vi "main.vi"() -> ()   [LabVIEW 2018]
uses:
  D:/NI LabVIEW/PowerControlWithAT2/REMOTE_SEE_CONTROLLER/RemoteSeeAbleService.dll
  RemoteSeeAbleService.dll
panel:
  in  "TryParrySeeDone":bool
  in  "StartTryParrySee":bool
  in  "ShutdownDone":bool
  in  "StartShutdown":bool
  in  "IsParryable":bool
  in  "ExamineSeeDone":bool
  in  "StartExamineSee":bool
  in  "stop":bool
  in  "CheckSeeDone":bool
  in  "StartCheckSee":bool
  in  "SeeInfo":string
  in  "IsIncomplete":bool
  in  "IsSee":bool
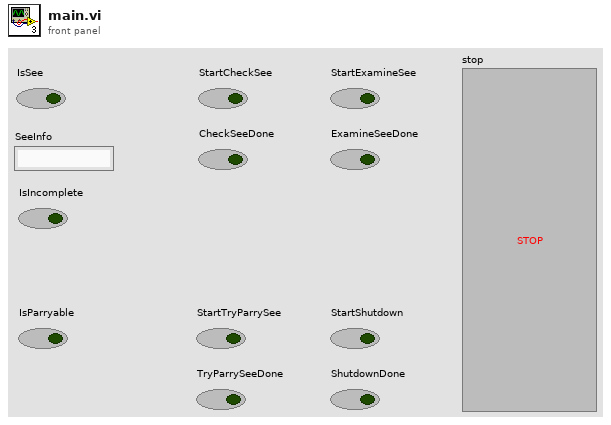
[diagram p1: front panel]
types:
  T1 = cluster{"StartCheckSee":refnum<vi>, "CheckSeeDone":refnum<vi>, "IsSee":refnum<vi>, "SeeInfo":refnum<vi>, "IsIncomplete":refnum<vi>}
  T2 = cluster{"StartExamineSee":refnum<vi>, "ExamineSeeDone":refnum<vi>, "IsSee":refnum<vi>, "SeeInfo":refnum<vi>, "IsIncomplete":refnum<vi>}
  T3 = cluster{"StartShutdown":refnum<vi>, "ShutdownDone":refnum<vi>}
  T4 = cluster{"StartTryParrySee":refnum<vi>, "TryParrySeeDone":refnum<vi>}
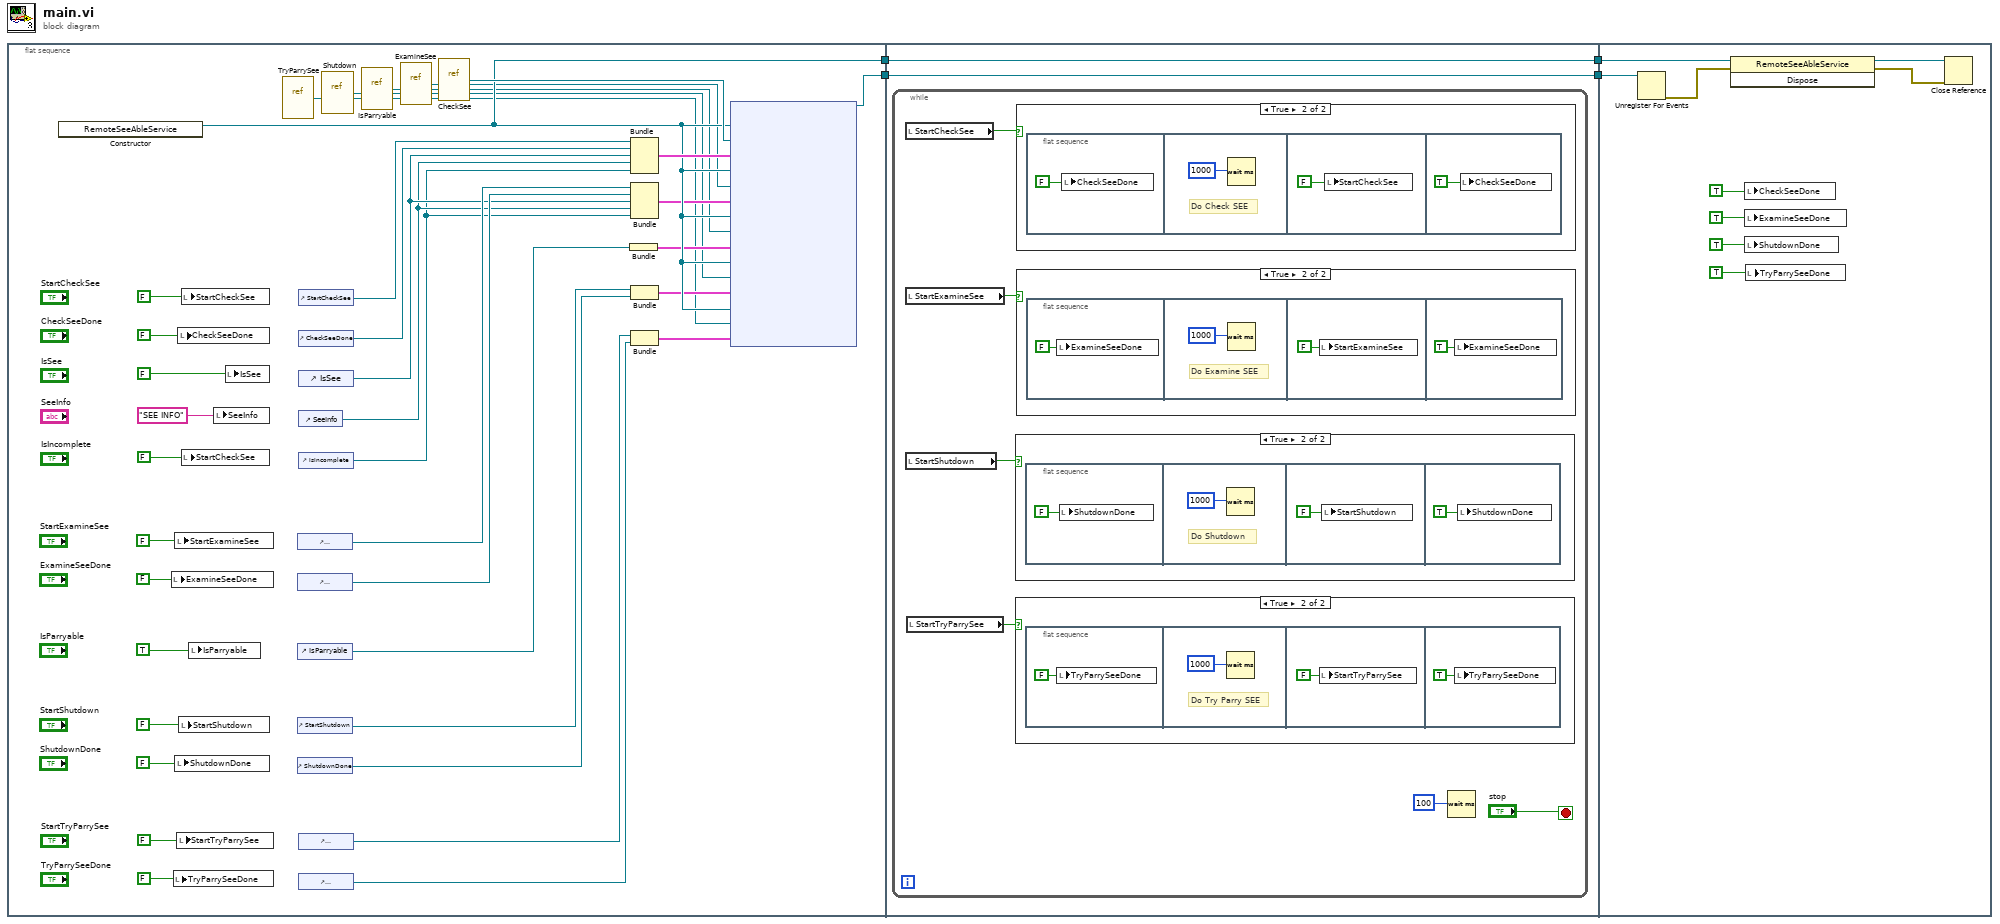
[diagram p0: block diagram]
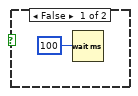
[diagram p2: hidden frame]
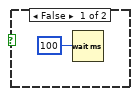
[diagram p3: hidden frame]
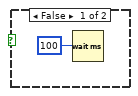
[diagram p4: hidden frame]
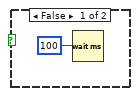
[diagram p5: hidden frame]
diagram:
  n1 = flat-sequence {
    tunnel: [w31] -> w3
    tunnel: [w30] -> w1
    tunnel: [w42] -> w4
    tunnel: w3 -> [w42]
    tunnel: [w41] -> w2
    tunnel: w1 -> [w41]
    tunnel: w4 -> [w76]
    tunnel: w2 -> [w75]
    frame #0 {
      n2 = constructor class="RemoteSeeAbleService"() -> (reference out=w31:refnum<k24>)  [unwired: 3 in, 2 out]
      n3 = local write "ExamineSeeDone"(FALSE ("StartCheckSee")) -> ()
      n4 = local write "TryParrySeeDone"(FALSE ("StartCheckSee")) -> ()
      n5 = local write "StartExamineSee"(FALSE ("StartCheckSee")) -> ()
      n6 = local write "ShutdownDone"(FALSE ("StartCheckSee")) -> ()
      n7 = local write "StartTryParrySee"(FALSE ("StartCheckSee")) -> ()
      n8 = local write "CheckSeeDone"(FALSE ("StartCheckSee")) -> ()
      n9 = local write "StartShutdown"(FALSE ("StartCheckSee")) -> ()
      n10 = local write "StartCheckSee"(FALSE ("StartCheckSee")) -> ()
      n11 = local write "StartCheckSee"(FALSE ("StartCheckSee")) -> ()
      n12 = local write "IsParryable"(TRUE ("StartCheckSee")) -> ()
      n13 = local write "SeeInfo"("SEE INFO" ("SeeInfo")) -> ()
      n14 = local write "IsSee"(FALSE ("StartCheckSee")) -> ()
      n15 = vi-ref "TryParrySee.vi"() -> ("vi reference"=w5:refnum<vi>)
      n16 = control-ref of="StartExamineSee"() -> (w27:refnum<vi>)
      n17 = control-ref of="ExamineSeeDone"() -> (w26:refnum<vi>)
      n18 = control-ref of="IsParryable"() -> (w20:refnum<vi>)
      n19 = control-ref of="StartShutdown"() -> (w16:refnum<vi>)
      n20 = control-ref of="ShutdownDone"() -> (w15:refnum<vi>)
      n21 = control-ref of="StartCheckSee"() -> (w39:refnum<vi>)
      n22 = control-ref of="CheckSeeDone"() -> (w38:refnum<vi>)
      n23 = control-ref of="IsSee"() -> (w25:refnum<vi>)
      n24 = control-ref of="SeeInfo"() -> (w24:refnum<vi>)
      n25 = control-ref of="IsIncomplete"() -> (w23:refnum<vi>)
      n26 = control-ref of="StartTryParrySee"() -> (w11:refnum<vi>)
      n27 = control-ref of="TryParrySeeDone"() -> (w10:refnum<vi>)
      n28 = vi-ref "Shutdown.vi"() -> ("vi reference"=w6:refnum<vi>)
      n29 = vi-ref "IsParryable.vi"() -> ("vi reference"=w7:refnum<vi>)
      n30 = vi-ref "ExamineSee.vi"() -> ("vi reference"=w8:refnum<vi>)
      n31 = vi-ref "CheckSee.vi"() -> ("vi reference"=w37:refnum<vi>)
      n32 = Bundle("IsParryable"=w20) -> (w19:cluster{"IsParryable":refnum<vi>})  [unwired: 1 in]
      n33 = Bundle("StartCheckSee"=w39, "CheckSeeDone"=w38, "IsSee"=w25, "SeeInfo"=w24, "IsIncomplete"=w23) -> (w40:T1)  [unwired: 1 in]
      n34 = Bundle("StartExamineSee"=w27, "ExamineSeeDone"=w26, "IsSee"=w25, "SeeInfo"=w24, "IsIncomplete"=w23) -> (w22:T2)  [unwired: 1 in]
      n35 = Bundle("StartShutdown"=w16, "ShutdownDone"=w15) -> (w14:T3)  [unwired: 1 in]
      n36 = Bundle("StartTryParrySee"=w11, "TryParrySeeDone"=w10) -> (w9:T4)  [unwired: 1 in]
      n37 = node(w31, w37, w40, w31, w8, w22, w31, w7, w19, w31, w6, w14, w31, w5, w9) -> (w30:refnum<k27>)  [unwired: 2 in, 1 out]
    }
    frame #1 {
      n38 = while {
        stop <- "stop" stop-if-true
        n39 = local read "StartCheckSee"() -> (w48:bool)
        n40 = local read "StartExamineSee"() -> (w45:bool)
        n41 = local read "StartShutdown"() -> (w44:bool)
        n42 = local read "StartTryParrySee"() -> (w43:bool)
        n43 = case shown="True" w44 {
          frame False {
            n44 = Wait (ms)(milliseconds to wait=u32 100) -> ()  [unwired: 1 out]
          }
          frame True {
            n45 = flat-sequence {
              frame #0 {
                n46 = local write "ShutdownDone"(FALSE ("StartCheckSee")) -> ()
              }
              frame #1 {
                # "Do Shutdown"
                n47 = Wait (ms)(milliseconds to wait=u32 1000) -> ()  [unwired: 1 out]
              }
              frame #2 {
                n48 = local write "StartShutdown"(FALSE ("StartCheckSee")) -> ()
              }
              frame #3 {
                n49 = local write "ShutdownDone"(TRUE ("StartCheckSee")) -> ()
              }
            }
          }
        }
        n50 = case shown="True" w43 {
          frame False {
            n51 = Wait (ms)(milliseconds to wait=u32 100) -> ()  [unwired: 1 out]
          }
          frame True {
            n52 = flat-sequence {
              frame #0 {
                n53 = local write "TryParrySeeDone"(FALSE ("StartCheckSee")) -> ()
              }
              frame #1 {
                # "Do Try Parry SEE"
                n54 = Wait (ms)(milliseconds to wait=u32 1000) -> ()  [unwired: 1 out]
              }
              frame #2 {
                n55 = local write "StartTryParrySee"(FALSE ("StartCheckSee")) -> ()
              }
              frame #3 {
                n56 = local write "TryParrySeeDone"(TRUE ("StartCheckSee")) -> ()
              }
            }
          }
        }
        n57 = case shown="True" w48 {
          frame False {
            n58 = Wait (ms)(milliseconds to wait=u32 100) -> ()  [unwired: 1 out]
          }
          frame True {
            n59 = flat-sequence {
              frame #0 {
                n60 = local write "CheckSeeDone"(FALSE ("StartCheckSee")) -> ()
              }
              frame #1 {
                # "Do Check SEE"
                n61 = Wait (ms)(milliseconds to wait=u32 1000) -> ()  [unwired: 1 out]
              }
              frame #2 {
                n62 = local write "StartCheckSee"(FALSE ("StartCheckSee")) -> ()
              }
              frame #3 {
                n63 = local write "CheckSeeDone"(TRUE ("StartCheckSee")) -> ()
              }
            }
          }
        }
        n64 = case shown="True" w45 {
          frame False {
            n65 = Wait (ms)(milliseconds to wait=u32 100) -> ()  [unwired: 1 out]
          }
          frame True {
            n66 = flat-sequence {
              frame #0 {
                n67 = local write "ExamineSeeDone"(FALSE ("StartCheckSee")) -> ()
              }
              frame #1 {
                # "Do Examine SEE"
                n68 = Wait (ms)(milliseconds to wait=u32 1000) -> ()  [unwired: 1 out]
              }
              frame #2 {
                n69 = local write "StartExamineSee"(FALSE ("StartCheckSee")) -> ()
              }
              frame #3 {
                n70 = local write "ExamineSeeDone"(TRUE ("StartCheckSee")) -> ()
              }
            }
          }
        }
        n71 = Wait (ms)(milliseconds to wait=u32 100) -> ()  [unwired: 1 out]
      }
    }
    frame #2 {
      n72 = Unregister For Events(event registration refnum=w75) -> (error out=w74:errorcluster)  [unwired: 1 in]
      n73 = invoke class="RemoteSeeAbleService" method="Dispose"(reference=w76, error in=w74) -> (reference out=w73:refnum<k24>, error out=w72:errorcluster)  [unwired: 1 in, 1 out]
      n74 = local write "CheckSeeDone"(TRUE ("StartCheckSee")) -> ()
      n75 = local write "ExamineSeeDone"(TRUE ("StartCheckSee")) -> ()
      n76 = local write "ShutdownDone"(TRUE ("StartCheckSee")) -> ()
      n77 = local write "TryParrySeeDone"(TRUE ("StartCheckSee")) -> ()
      n78 = Close Reference(reference=w73, error in (no error)=w72) -> ()  [unwired: 1 out]
    }
  }
